vi "Process Clock.vi"(10 "EEPROM in":refnum<class "EEPROM.lvclass">, 11 "IO in":refnum<class "IO.lvclass">) -> (2 "EEPROM out":refnum<class "EEPROM.lvclass">, 3 "IO out":refnum<class "IO.lvclass">)   [LabVIEW 2021, in "IO.lvclass"]
uses:
  IO.lvclass
  EEPROM/EEPROM.lvclass
  IO.lvclass/IO.ctl
  EEPROM/EEPROM.lvclass/EEPROM.ctl
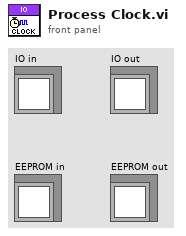
[diagram p1: front panel]
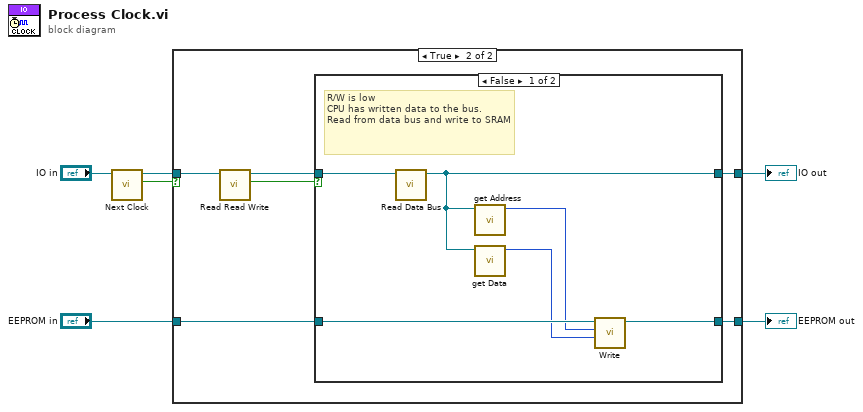
[diagram p0: block diagram]
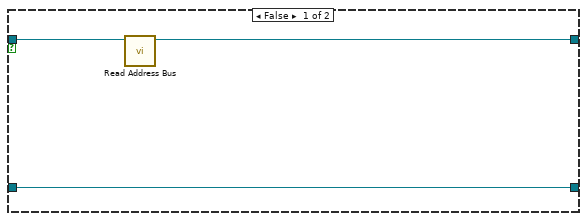
[diagram p2: hidden frame]
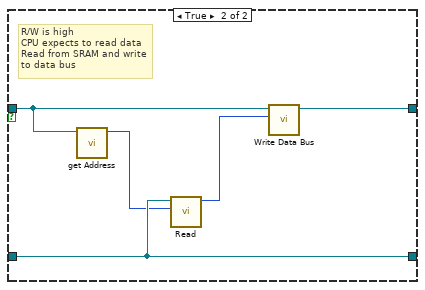
[diagram p3: hidden frame]
diagram:
  n1 = call "Next Clock.vi"("Clock Generator in"="IO in") -> ("Current State"=w4:bool, "Clock Generator out"=w5:refnum<class "IO.lvclass">)  [unwired: 8 in, 1 out]
  n2 = case shown="True" w4 {
    tunnel: [w9 w14] -> w1
    tunnel: "EEPROM in" -> [w9 w15]
    tunnel: w5 -> [w8 w11]
    tunnel: [w7 w13] -> w6
    frame False {
      n3 = call "Read Address Bus.vi"("IO in"=w8) -> ("IO out"=w7:refnum<class "IO.lvclass">)  [unwired: 9 in, 1 out]
    }
    frame True {
      n4 = call "Read Read Write.vi"("IO in"=w11) -> ("R/W"=w10:bool, "IO out"=w12:refnum<class "IO.lvclass">)  [unwired: 8 in, 1 out]
      n5 = case shown="False" w10 {
        tunnel: w15 -> [w19 w24]
        tunnel: [w20 w24] -> w14
        tunnel: w12 -> [w21 w25]
        tunnel: [w16 w26] -> w13
        frame False {
          # "R/W is low\nCPU has written data to the bus. \nRead from data bus and write to SRAM"
          n6 = call "Read Data Bus.vi"("IO in"=w21) -> ("IO out"=w16:refnum<class "IO.lvclass">)  [unwired: 9 in, 1 out]
          n7 = call "get Address.vi"("IO in"=w16) -> ("Address"=w18:u16)  [unwired: 10 in]
          n8 = call "get Data.vi"("IO in"=w16) -> ("Data"=w17:u8)  [unwired: 10 in]
          n9 = call "Write.vi"("Data"=w17, "Address"=w18, "EEPROM in"=w19) -> ("EEPROM out"=w20:refnum<class "EEPROM.lvclass">)  [unwired: 8 in]
        }
        frame True {
          # "R/W is high\nCPU expects to read data\nRead from SRAM and write to data bus"
          n10 = call "get Address.vi"("IO in"=w25) -> ("Address"=w23:u16)  [unwired: 10 in]
          n11 = call "Read.vi"("Address"=w23, "EEPROM in"=w24) -> ("Data"=w22:u8)  [unwired: 9 in]
          n12 = call "Write Data Bus.vi"("Data"=w22, "IO in"=w25) -> ("IO out"=w26:refnum<class "IO.lvclass">)  [unwired: 8 in, 1 out]
        }
      }
    }
  }
  "IO out" <- w6
  "EEPROM out" <- w1
